vi "array_mem_operation2.vi"() -> ()   [LabVIEW 2019]
uses:
  <vilib>/Analysis/1siggen.llb/General Aperiodic Triangle.vi
  <vilib>/Analysis/NI_AALBase.lvlib
panel:
  out "Waveform Graph":dbl[](graph)
  in  "stop":bool
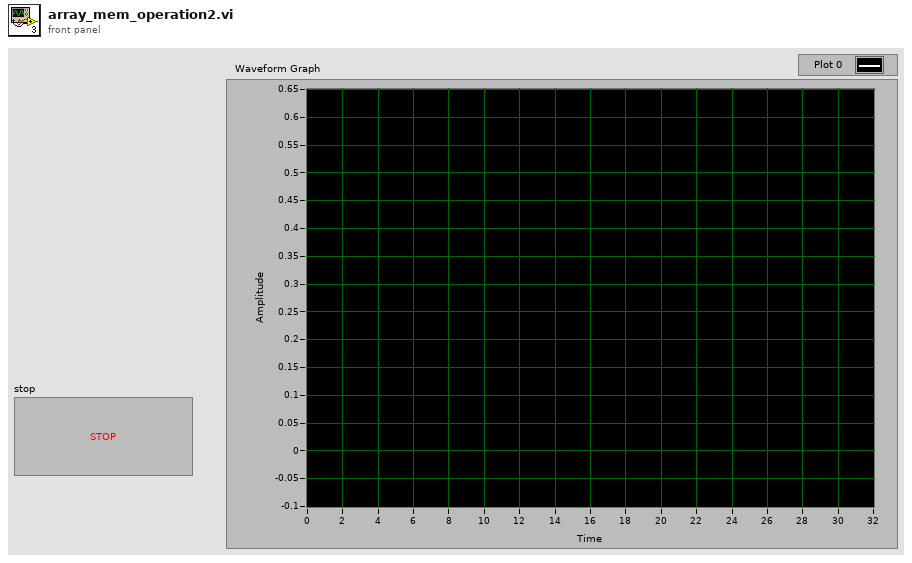
[diagram p1: front panel]
types:
  T1 = enum16{"open", "replace", "create", "open or create", "replace or create", "replace or create with confirmation"}
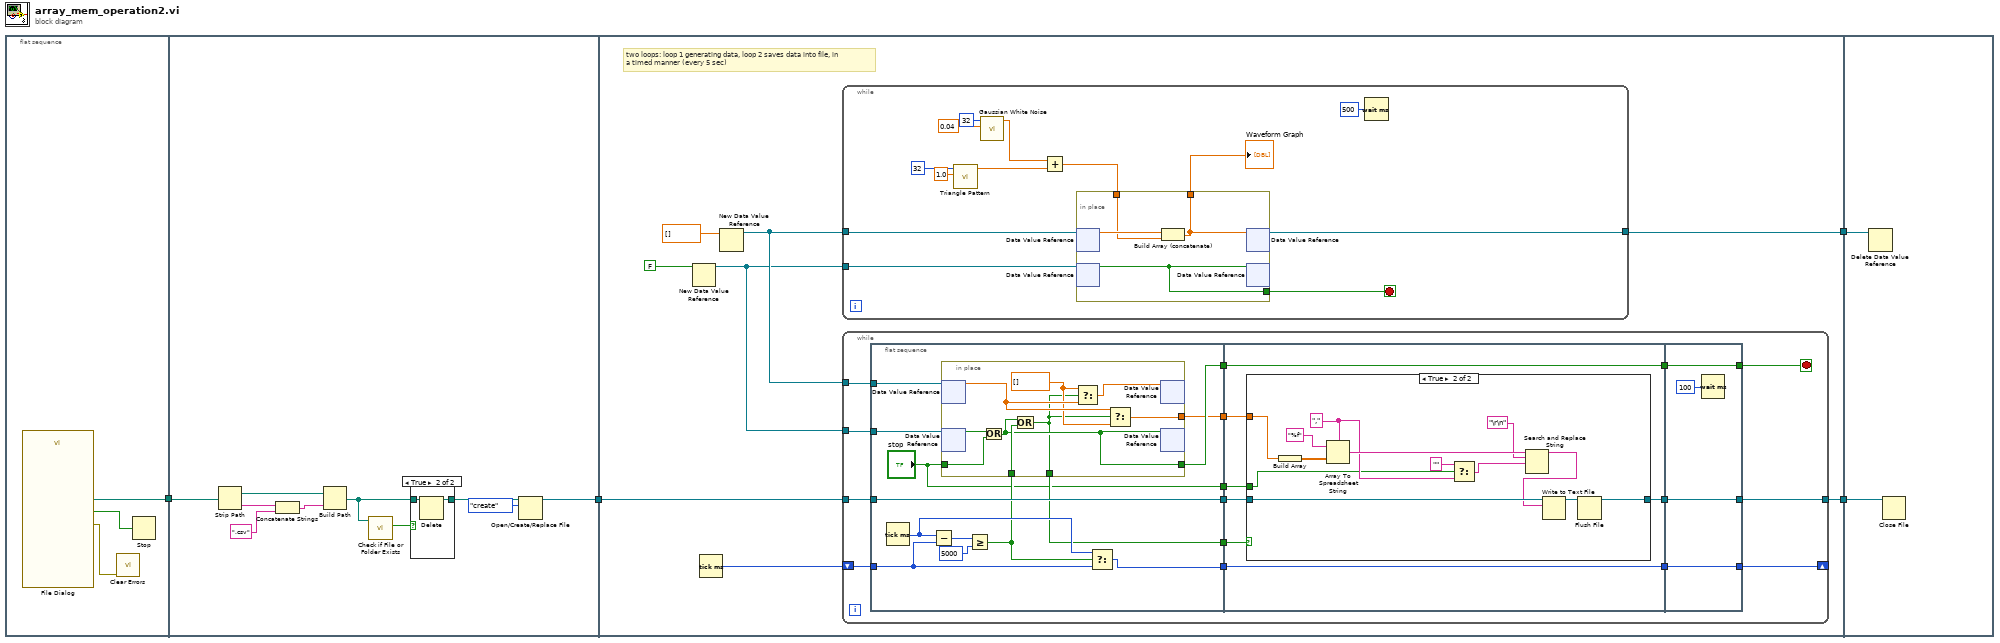
[diagram p0: block diagram]
diagram:
  n1 = flat-sequence {
    tunnel: [w5] -> w3
    tunnel: w3 -> [w17]
    tunnel: [w8] -> w2
    tunnel: [w26] -> w4
    tunnel: w2 -> [w22]
    tunnel: [w21] -> w1
    tunnel: w4 -> [w110]
    tunnel: w1 -> [w109]
    frame #0 {
      n2 = call "File Dialog"() -> ("selected path"=w5:path, "cancelled"=w7:bool, "error out"=w6:errorcluster)  [unwired: 12 in, 1 out]
      n3 = call <vilib>:"Clear Errors.vi"("error in (no error)"=w6) -> ()  [unwired: 5 in, 2 out]
      n4 = Stop(stop? (T)=w7) -> ()
    }
    frame #1 {
      n5 = Strip Path(path=w17) -> (stripped path=w14:path, name=w16:string)
      n6 = Concatenate Strings(w16, ".csv") -> (w13:string)
      n7 = Build Path(base path=w14, name or relative path=w13) -> (appended path=w11:path)
      n8 = call <vilib>:"Check if File or Folder Exists.vi"("path"=w11) -> ("file or folder exists?"=w12:bool)  [unwired: 8 in, 2 out]
      n9 = case shown="True" w12 {
        tunnel: w11 -> [w18 w20]
        tunnel: [w18 w19] -> w10
        frame False {
        }
        frame True {
          n10 = Delete(path (use dialog)=w20) -> (deleted path=w19:path)  [unwired: 4 in, 2 out]
        }
      }
      n11 = Open/Create/Replace File(file path (use dialog)=w10, operation (0:open)=T1."create") -> (refnum out=w8:refnum<file>)  [unwired: 4 in, 2 out]
    }
    frame #2 {
      # "two loops: loop 1 generating data, loop 2 saves data into file, in\na timed manner (every 5 sec)"
      n12 = New Data Value Reference(data value=FALSE) -> (data value reference=w24:refnum<data-value>)  [unwired: 1 in, 1 out]
      n13 = Tick Count (ms)() -> (millisecond timer value=w23:u32)
      n14 = New Data Value Reference(data value=dbl[] []) -> (data value reference=w27:refnum<data-value>)  [unwired: 1 in, 1 out]
      n15 = while {
        tunnel: w27 -> [w44]
        tunnel: w24 -> [w43]
        shift-right: [w36] -> _
        shift-left: w23 -> [w39]
        tunnel: w22 -> [w33]
        tunnel: [w30] -> w21
        stop <- w40 stop-if-true
        n16 = flat-sequence {
          tunnel: w44 -> [w57]
          tunnel: w43 -> [w56]
          tunnel: [w55] -> w42
          tunnel: w39 -> [w51]
          tunnel: [w50] -> w38
          tunnel: [w49] -> w35
          tunnel: [w46] -> w34
          tunnel: w33 -> [w48]
          tunnel: [w48] -> w32
          tunnel: ["stop"] -> w29
          tunnel: w42 -> [w73]
          tunnel: [w73] -> w41
          tunnel: w38 -> [w72]
          tunnel: [w72] -> w37
          tunnel: w35 -> [w70]
          tunnel: w34 -> [w71]
          tunnel: w32 -> [w69]
          tunnel: [w68] -> w31
          tunnel: w29 -> [w67]
          tunnel: w41 -> [w90]
          tunnel: [w90] -> w40
          tunnel: w37 -> [w89]
          tunnel: [w89] -> w36
          tunnel: w31 -> [w88]
          tunnel: [w88] -> w30
          frame #0 {
            n17 = Tick Count (ms)() -> (millisecond timer value=w52:u32)
            n18 = Subtract(x=w52, y=w51) -> (x-y=w54:u32)
            n19 = Greater Or Equal?(x=w54, y=5000) -> (x >= y?=w47:bool)
            n20 = in-place {
              in-place-border: [w59] -> w55
              in-place-border: [w64] -> w49
              in-place-border: "stop" -> [w63]
              in-place-border: w47 -> [w60]
              in-place-border: [w58] -> w46
              w61 = dbl[] [] ("t")
              n21 = in-place-dvr #1(w57) -> (w62:dbl[])  [unwired: 1 out]
              n22 = in-place-dvr #2(w56) -> (w66:bool)  [unwired: 1 out]
              n23 = Or(x=w66, y=w63) -> (x .or. y?=w59:bool)
              n24 = Or(x=w59, y=w60) -> (x .or. y?=w58:bool)
              n25 = Select(t=w61, s=w58, f=w62) -> (s? t:f=w65:dbl[])
              n26 = Select(t=w62, s=w58, f=w61) -> (s? t:f=w64:dbl[])
              n27 = in-place-dvr #1(w65) -> ()  [unwired: 2 out]
              n28 = in-place-dvr #2(w59) -> ()  [unwired: 2 out]
            }
            n29 = Select(t=w52, s=w47, f=w51) -> (s? t:f=w50:u32)
          }
          frame #1 {
            n30 = case shown="True" w71 {
              tunnel: w70 -> [_ w83]
              tunnel: w69 -> [w74 w87]
              tunnel: [w74 w85] -> w68
              tunnel: w67 -> [_ w76]
              frame False {
              }
              frame True {
                w78 = "," ("delimiter (Tab)")
                n31 = Build Array(w83) -> (w82:dbl[][])
                n32 = Array To Spreadsheet String(delimiter (Tab)=w78, array=w82, 3:"%f" ("format string")) -> (spreadsheet string=w81:string)
                n33 = Select(t="", s=w76, f=w78) -> (s? t:f=w77:string)
                n34 = Search and Replace String(input string=w81, search string="\r\n", replace string=w77) -> (result string=w80:string)  [unwired: 5 in, 3 out]
                n35 = Write to Text File(file (use dialog)=w87, text=w80) -> (refnum out=w86:refnum<file>)  [unwired: 2 in, 2 out]
                n36 = Flush File(refnum=w86) -> (refnum out=w85:refnum<file>)  [unwired: 1 in, 1 out]
              }
            }
          }
          frame #2 {
            n37 = Wait (ms)(milliseconds to wait=u32 100) -> ()  [unwired: 1 out]
          }
        }
      }
      n38 = while {
        tunnel: w27 -> [w98]
        tunnel: [w95] -> w26
        tunnel: w24 -> [w94]
        stop <- w93 stop-if-true
        n39 = call <vilib>:"Triangle Pattern.vi"("amplitude"=1.0, "samples"=32) -> ("Triangle Pattern"=w99:dbl[])  [unwired: 8 in, 1 out]
        n40 = call <vilib>:"Gaussian White Noise.vi"("standard deviation"=0.04, "samples"=32) -> ("Gaussian noise pattern"=w100:dbl[])  [unwired: 8 in, 1 out]
        n41 = Add(x=w100, y=w99) -> (x+y=w96:dbl[])
        n42 = in-place {
          in-place-border: w96 -> [w107]
          in-place-border: [w106] -> w93
          in-place-border: [w105] -> w92
          n43 = in-place-dvr #3(w98) -> (w108:dbl[])  [unwired: 1 out]
          n44 = in-place-dvr #4(w94) -> (w106:bool)  [unwired: 1 out]
          n45 = Build Array (concatenate)(w108, w107) -> (w105:dbl[])
          n46 = in-place-dvr #3(w105) -> (w95:refnum<data-value>)  [unwired: 1 out]
          n47 = in-place-dvr #4(w106) -> ()  [unwired: 2 out]
        }
        "Waveform Graph" <- w92
        n48 = Wait (ms)(milliseconds to wait=u32 500) -> ()  [unwired: 1 out]
      }
    }
    frame #3 {
      n49 = Delete Data Value Reference(data value reference=w110) -> ()  [unwired: 1 in, 2 out]
      n50 = Close File(refnum=w109) -> ()  [unwired: 1 in, 2 out]
    }
  }
